vi "AcceptDriverError.vi"(8 "error in (no error)":errorcluster, 11 "status":i32) -> (0 "error out":errorcluster)   [LabVIEW 2020, in "NI_TargetHelper.lvlib"]
uses:
  <vilib>/TargetSupport/NI_TargetHelper/NI_TargetHelper.lvlib
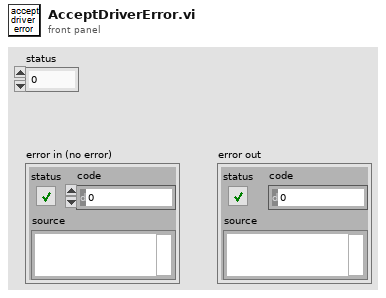
[diagram p1: front panel]
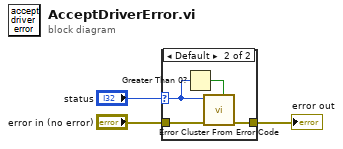
[diagram p0: block diagram]
diagram:
  n1 = case shown="Default" "status" {
    selector: "status" -> [_ w5]
    tunnel: [w4 w7] -> w3
    tunnel: "error in (no error)" -> [w4 w8]
    frame 0 {
    }
    frame Default {
      n2 = Greater Than 0?(x=w5) -> (x > 0?=w6:bool)
      n3 = call <vilib>:"Error Cluster From Error Code.vi"("is warning? (False)"=w6, "error in (no error)"=w8, "error code (0)"=w5) -> ("error out"=w7:errorcluster)  [unwired: 6 in]
    }
  }
  "error out" <- w3
